vi "ultrasonic.vi"() -> ()   [LabVIEW 2022 SP3]
uses:
  <vilib>/DAQmx/read.llb/DAQmx Read (Analog Wfm 1Chan NSamp).vi
  <vilib>/DAQmx/write.llb/DAQmx Write (Digital Bool 1Line 1Point).vi
  <vilib>/DAQmx/create/channels.llb/DAQmx Create Channel (DO-Digital Output).vi
  <vilib>/DAQmx/miscellaneous.llb/DAQmx Fill In Error Info.vi
  <vilib>/DAQmx/create/channels.llb/DAQmx Create Channel (AI-Voltage-Basic).vi
  <vilib>/DAQmx/configure/timing.llb/DAQmx Timing (Sample Clock).vi
  Global distance.vi
panel:
  out "Distance":dbl format="%#_3g"
  out "Waveform Graph":waveform(dbl)(graph)
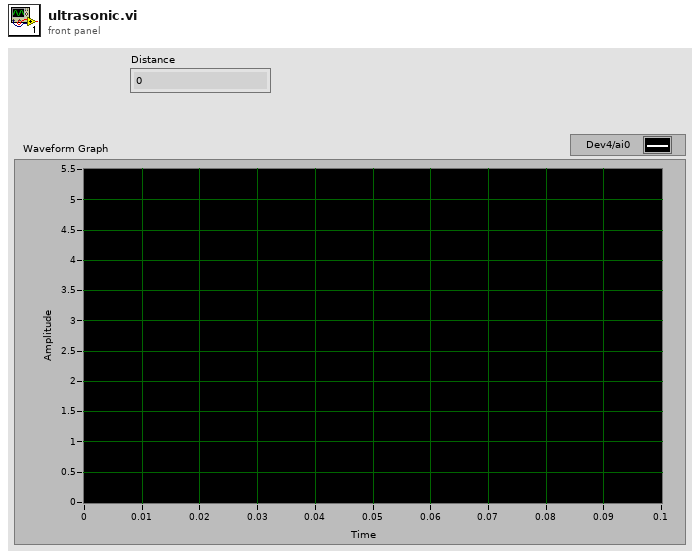
[diagram p1: front panel]
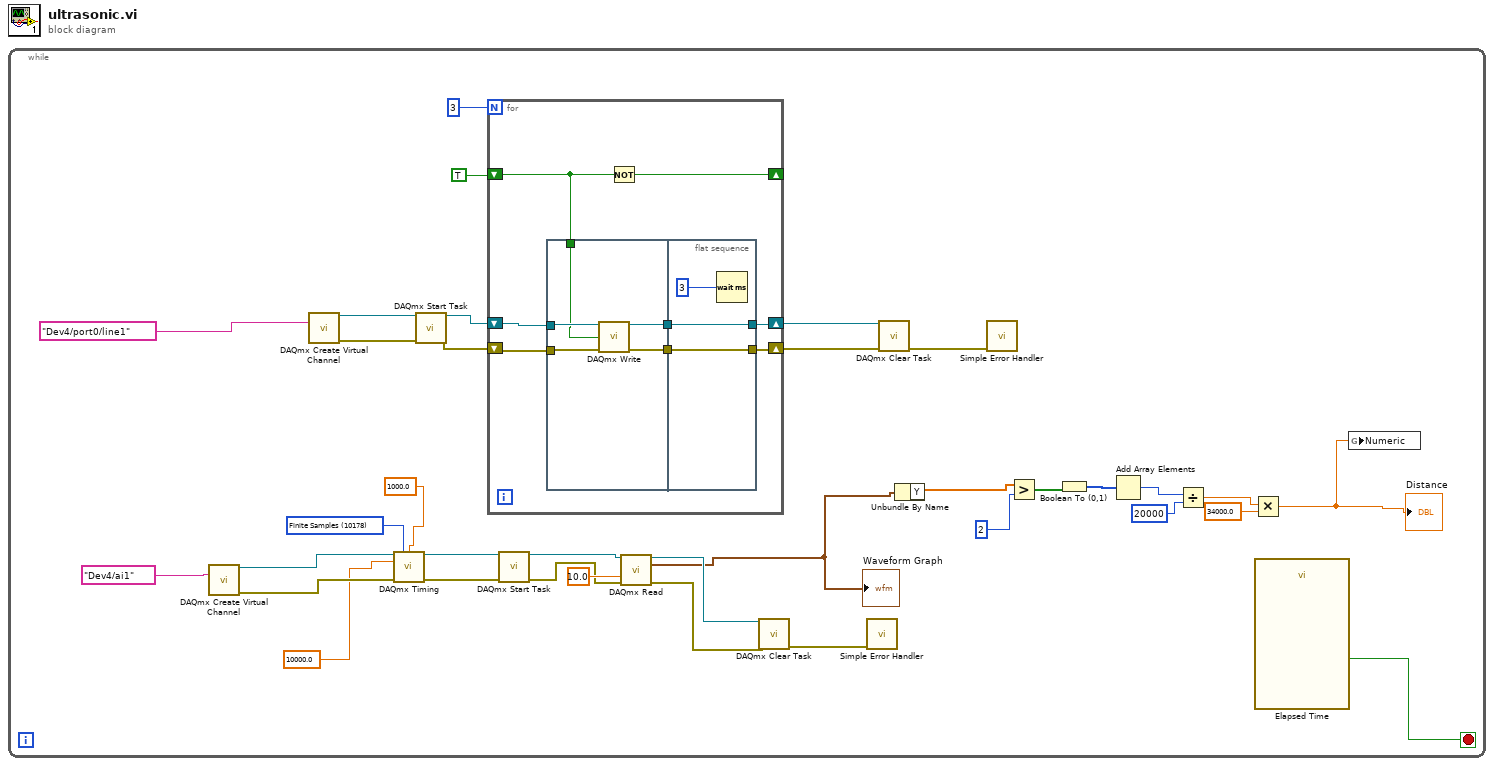
[diagram p0: block diagram]
diagram:
  n1 = while {
    stop <- w1 stop-if-true
    w26 = 10178 items=["Finite Samples"=10178, "Continuous Samples"=10123, "Hardware Timed Single Point"=12522] ("sample mode")
    n2 = call-poly <vilib>:"DAQmx Create Virtual Channel.vi"("physical channels"=tag "Dev4/ai1" ("DAQmx Physical Channel 2")) -> ("task out"=w25:refnum<k21>, "error out"=w24:errorcluster)  [unwired: 13 in]
    n3 = call-poly <vilib>:"DAQmx Create Virtual Channel.vi"("lines"=tag "Dev4/port0/line1" ("DAQmx Physical Channel")) -> ("task out"=w35:refnum<k21>, "error out"=w34:errorcluster)  [unwired: 13 in]
    n4 = call-poly <vilib>:"DAQmx Timing.vi"("task/channels in"=w25, "sample mode"=w26, "samples per channel"=1000.0 ("Number of samples"), "rate"=10000.0 ("Sampling frequency"), "error in"=w24) -> ("task out"=w23:refnum<k21>, "error out"=w22:errorcluster)  [unwired: 9 in]
    n5 = call <vilib>:"DAQmx Start Task.vi"("task/channels in"=w35, "error in"=w34) -> ("task out"=w33:refnum<k21>, "error out"=w32:errorcluster)  [unwired: 12 in]
    n6 = for {
      N: 3 -> [_]
      shift-right: [w39] -> w30
      shift-left: w33 -> [w41]
      shift-right: [w38] -> w29
      shift-left: w32 -> [w40]
      shift-right: [w37] -> _
      shift-left: TRUE -> [w36]
      n7 = flat-sequence {
        tunnel: w41 -> [w48]
        tunnel: w40 -> [w47]
        tunnel: [w46] -> w43
        tunnel: [w45] -> w42
        tunnel: w36 -> [w44]
        tunnel: [w50] -> w39
        tunnel: w43 -> [w50]
        tunnel: [w49] -> w38
        tunnel: w42 -> [w49]
        frame #0 {
          n8 = call-poly <vilib>:"DAQmx Write.vi"("task/channels in"=w48, "data"=w44, "error in"=w47) -> ("task out"=w46:refnum<k21>, "error out"=w45:errorcluster)  [unwired: 10 in, 1 out]
        }
        frame #1 {
          n9 = Wait (ms)(milliseconds to wait=u32 3) -> ()  [unwired: 1 out]
        }
      }
      n10 = Not(x=w36) -> (.not. x?=w37:bool)
    }
    n11 = call <vilib>:"DAQmx Start Task.vi"("task/channels in"=w23, "error in"=w22) -> ("task out"=w20:refnum<k21>, "error out"=w19:errorcluster)  [unwired: 12 in]
    n12 = call-poly <vilib>:"DAQmx Read.vi"("task/channels in"=w20, "timeout"=10.0, "error in"=w19) -> ("task out"=w14:refnum<k21>, "data"=w11:waveform(dbl), "error out"=w17:errorcluster)  [unwired: 10 in]
    "Waveform Graph" <- w11
    n13 = call <vilib>:"DAQmx Clear Task.vi"("task in"=w14, "error in"=w17) -> ("error out"=w18:errorcluster)  [unwired: 13 in]
    n14 = call <vilib>:"Simple Error Handler.vi"("error in (no error)"=w18) -> ()  [unwired: 4 in, 5 out]
    n15 = call <vilib>:"DAQmx Clear Task.vi"("task in"=w30, "error in"=w29) -> ("error out"=w31:errorcluster)  [unwired: 13 in]
    n16 = Unbundle By Name(w11) -> ("Y"=w12:dbl[])
    n17 = call <vilib>:"Simple Error Handler.vi"("error in (no error)"=w31) -> ()  [unwired: 4 in, 5 out]
    n18 = Greater?(x=w12, y=2) -> (0:w10:bool[])
    n19 = Boolean To (0,1)(Boolean=w10) -> (0, 1=w9:i16[])
    n20 = Add Array Elements(numeric array=w9) -> (sum=w5:i16)
    n21 = Divide(x=w5, y=i16 20000) -> (x/y=w6:dbl)
    n22 = Multiply(x=w6, y=34000.0) -> (x*y=w2:dbl)
    "Distance" <- w2
    n23 = call "Elapsed Time"() -> ("Time has Elapsed"=w1:bool)  [unwired: 12 in, 7 out]
    n24 = global write "Global distance.vi" "Numeric"(w2) -> ()
  }
